vi "Get_Joystick.vi"(1 "Joystick_One":string="Pilot Controller", 2 "Joystick_Two":string="CoPilot Controller") -> (6 "Joystick_Out":T1)   [LabVIEW 2019]
uses:
  Joystick_Controls.ctl
  <vilib>/Rock Robotics/WPI/Utilities/WPI_GetSetVariantRefNum.vi
  <vilib>/Rock Robotics/WPI/Joystick/WPI_JoystickDeviceEnum.ctl
panel:
  in  "Joystick Controls":T1
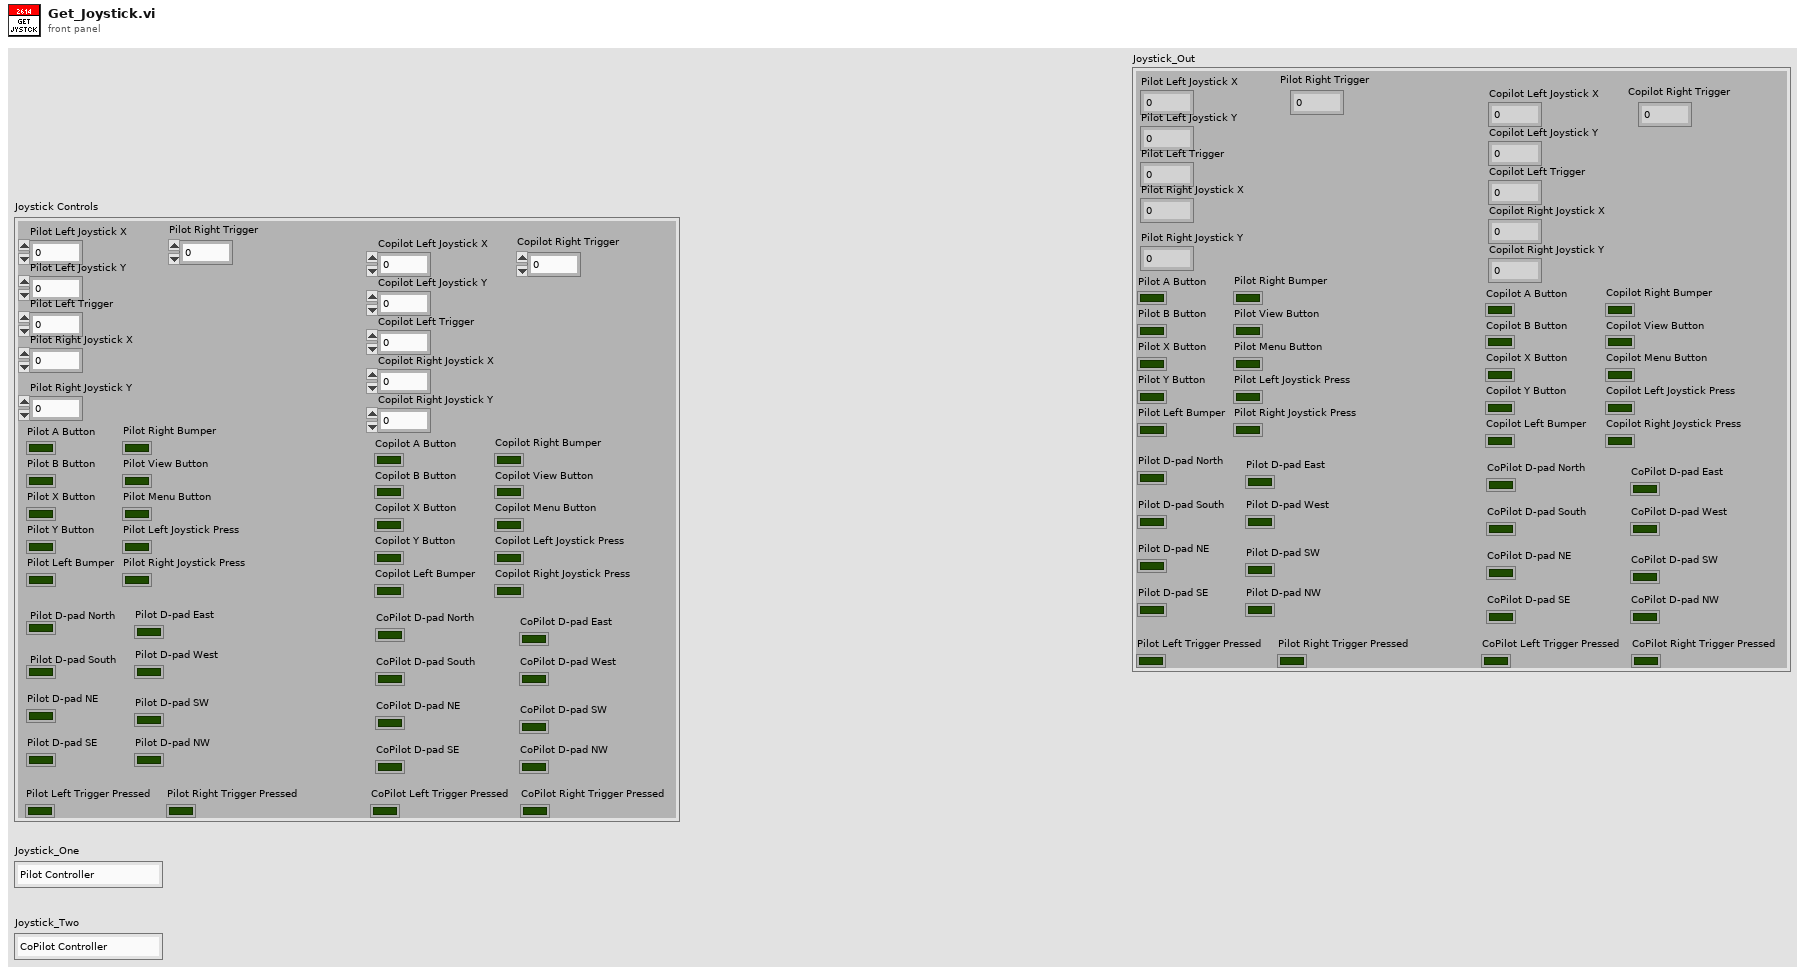
[diagram p1: front panel]
types:
  T1 = typedef "Joystick_Controls.ctl" = cluster{"Pilot Left Joystick X":dbl, "Pilot Left Joystick Y":dbl, "Pilot A Button":bool, "Pilot B Button":bool, "Pilot X Button":bool, "Pilot Y Button":bool, "Pilot Left Bumper":bool, "Pilot Right Bumper":bool, "Pilot View Button":bool, "Pilot Menu Button":bool, "Pilot Left Joystick Press":bool, "Pilot Right Joystick Press":bool, "Pilot Left Trigger":dbl, "Pilot Right Joystick X":dbl, "Pilot Right Joystick Y":dbl, "Pilot Right Trigger":dbl, "Copilot Left Joystick X":dbl, "Copilot Left Joystick Y":dbl, "Copilot A Button":bool, "Copilot B Button":bool, "Copilot X Button":bool, "Copilot Y Button":bool, "Copilot Left Bumper":bool, "Copilot Right Bumper":bool, "Copilot View Button":bool, "Copilot Menu Button":bool, "Copilot Left Joystick Press":bool, "Copilot Right Joystick Press":bool, "Copilot Left Trigger":dbl, "Copilot Right Joystick X":dbl, "Copilot Right Joystick Y":dbl, "Copilot Right Trigger":dbl, "Pilot D-pad North":bool, "Pilot D-pad South":bool, "Pilot D-pad East":bool, "Pilot D-pad West":bool, "Pilot D-pad NE ":bool, "Pilot D-pad SE":bool, "Pilot D-pad SW":bool, "Pilot D-pad NW":bool, "CoPilot D-pad North":bool, "CoPilot D-pad South":bool, "CoPilot D-pad East":bool, "CoPilot D-pad West":bool, "CoPilot D-pad NE":bool, "CoPilot D-pad SE":bool, "CoPilot D-pad SW":bool, "CoPilot D-pad NW":bool, "Pilot Left Trigger Pressed":bool, "Pilot Right Trigger Pressed":bool, "CoPilot Left Trigger Pressed":bool, "CoPilot Right Trigger Pressed":bool}
  T2 = typedef "WPI_JoystickDeviceEnum.ctl" = enum16{"USB 0", "USB 1", "USB 2", "USB 3", "USB 4", "USB 5"}
  T3 = typedef "WPI_Joystick Info.ctl" = cluster{"Device Name":string, "HID Type":T4, "XBox Type":T5, "Axes Count":i32, "Axes Types":T6[], "Button Count":i32, "POV Count":i32}
  T4 = typedef "WPI_JoystickHID Types.ctl" = enum16{"Not HID", "HID Joystick", "HID Gamepad", "HID Driving Wheel", "HID Flightstick", "HID First Person"}
  T5 = typedef "WPI_JoystickXBox Types.ctl" = enum16{"Not XBox", "XBox Unknown", "XBox Gamepad", "XBox Wheel", "XBox Arcade Stick", "XBox Flight Stick", "XBox Dance Pad", "XBox Guitar", "XBox Drum Kit", "XBox Arcade Pad"}
  T6 = typedef "WPI_JoystickAxis Types.ctl" = enum16{"X Axis", "Y Axis", "Z Axis", "RxAxis", "RyAxis", "RzAxis", "Slider", "POV", "None", "L X Axis", "L Y Axis", "L Trigger", "R Trigger", "R X Axis", "R Y Axis"}
  T7 = typedef "WPI_JoystickDevRef.ctl" = cluster{"Device":T2}
  T8 = cluster{"Axes[0]":dbl, "Axes[1]":dbl, "Axes[2]":dbl, "Axes[3]":dbl, "Axes[4]":dbl, "Axes[5]":dbl, "Axes[6]":dbl, "Axes[7]":dbl, "Axes[8]":dbl}
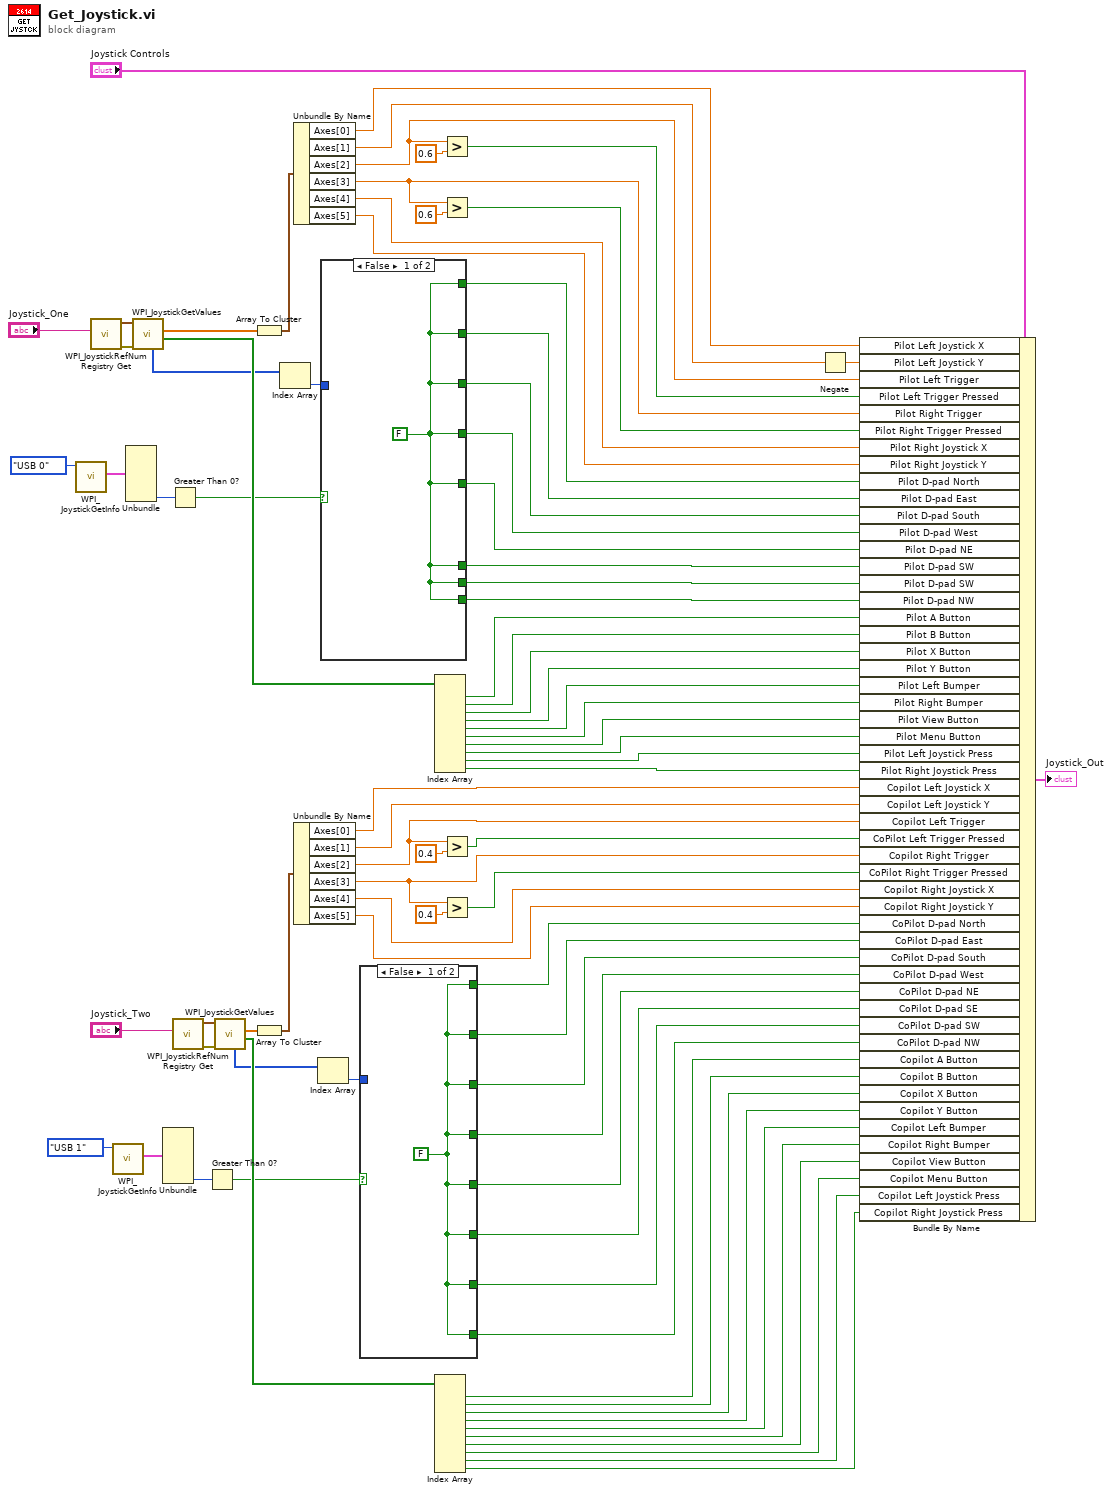
[diagram p0: block diagram]
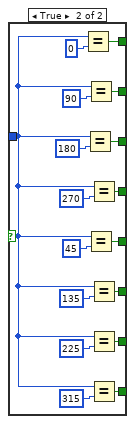
[diagram p2: hidden frame]
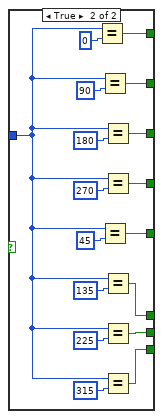
[diagram p3: hidden frame]
diagram:
  n1 = call <vilib>:"WPI_JoystickGetInfo.vi"("JoystickDevice"=WPI_JoystickDeviceEnum."USB 0") -> ("Joystick Info"=w7:T3)  [unwired: 9 in, 1 out]
  n2 = call <vilib>:"WPI_JoystickRefNum Registry Get.vi"("refnum name"="Joystick_One") -> ("error out"=w44:errorcluster, "JoystickDevRef"=w83:T7)  [unwired: 9 in]
  n3 = call <vilib>:"WPI_JoystickGetInfo.vi"("JoystickDevice"=WPI_JoystickDeviceEnum."USB 1") -> ("Joystick Info"=w3:T3)  [unwired: 9 in, 1 out]
  n4 = Unbundle(w7) -> ("POV Count"=w6:i32)  [unwired: 6 out]
  n5 = call <vilib>:"WPI_JoystickGetValues.vi"("error in (no error)"=w44, "JoystickDevRef"=w83) -> ("Buttons"=w76:bool[], "Axes"=w82:dbl[], "POVs"=w46:i16[])  [unwired: 5 in, 2 out]
  n6 = Unbundle(w3) -> ("POV Count"=w2:i32)  [unwired: 6 out]
  n7 = Greater Than 0?(x=w6) -> (x > 0?=w5:bool)
  n8 = call <vilib>:"WPI_JoystickRefNum Registry Get.vi"("refnum name"="Joystick_Two") -> ("error out"=w43:errorcluster, "JoystickDevRef"=w65:T7)  [unwired: 9 in]
  n9 = Greater Than 0?(x=w2) -> (x > 0?=w1:bool)
  n10 = call <vilib>:"WPI_JoystickGetValues.vi"("error in (no error)"=w43, "JoystickDevRef"=w65) -> ("Buttons"=w63:bool[], "Axes"=w64:dbl[], "POVs"=w45:i16[])  [unwired: 5 in, 2 out]
  n11 = Array To Cluster(array=w82) -> (cluster=w81:T8)
  n12 = Array To Cluster(array=w64) -> (cluster=w62:T8)
  n13 = Index Array(array=w46) -> (element=w33:i16)  [unwired: 1 in]
  n14 = Unbundle By Name(w81) -> ("Axes[0]"=w80:dbl, "Axes[1]"=w79:dbl, "Axes[2]"=w23:dbl, "Axes[3]"=w19:dbl, "Axes[4]"=w78:dbl, "Axes[5]"=w77:dbl)
  n15 = Unbundle By Name(w62) -> ("Axes[0]"=w61:dbl, "Axes[1]"=w60:dbl, "Axes[2]"=w16:dbl, "Axes[3]"=w13:dbl, "Axes[4]"=w59:dbl, "Axes[5]"=w58:dbl)
  n16 = Index Array(array=w45) -> (element=w24:i16)  [unwired: 1 in]
  n17 = case shown="False" w5 {
    tunnel: [w84 w101] -> w40
    tunnel: [w84 w100] -> w39
    tunnel: [w84 w99] -> w38
    tunnel: [w84 w98] -> w37
    tunnel: [w84 w97] -> w36
    tunnel: [w84 w96] -> w35
    tunnel: [w84 w95] -> w34
    tunnel: w33 -> [_ w85]
    tunnel: [w84 w86] -> w10
    frame False {
      w84 = FALSE
    }
    frame True {
      n18 = Equal?(x=w85, y=i16 0) -> (x = y?=w86:bool)
      n19 = Equal?(x=w85, y=i16 90) -> (x = y?=w101:bool)
      n20 = Equal?(x=w85, y=i16 45) -> (x = y?=w97:bool)
      n21 = Equal?(x=w85, y=i16 180) -> (x = y?=w100:bool)
      n22 = Equal?(x=w85, y=i16 270) -> (x = y?=w99:bool)
      n23 = Equal?(x=w85, y=i16 135) -> (x = y?=w96:bool)
      n24 = Equal?(x=w85, y=i16 225) -> (x = y?=w95:bool)
      n25 = Equal?(x=w85, y=i16 315) -> (x = y?=w98:bool)
    }
  }
  n26 = case shown="False" w1 {
    tunnel: [w102 w111] -> w32
    tunnel: [w102 w110] -> w31
    tunnel: [w102 w103] -> w30
    tunnel: [w102 w109] -> w29
    tunnel: [w102 w108] -> w28
    tunnel: [w102 w107] -> w27
    tunnel: [w102 w106] -> w26
    tunnel: [w102 w105] -> w25
    tunnel: w24 -> [_ w104]
    frame False {
      w102 = FALSE
    }
    frame True {
      n27 = Equal?(x=w104, y=i16 0) -> (x = y?=w111:bool)
      n28 = Equal?(x=w104, y=i16 180) -> (x = y?=w103:bool)
      n29 = Equal?(x=w104, y=i16 90) -> (x = y?=w110:bool)
      n30 = Equal?(x=w104, y=i16 45) -> (x = y?=w108:bool)
      n31 = Equal?(x=w104, y=i16 270) -> (x = y?=w109:bool)
      n32 = Equal?(x=w104, y=i16 135) -> (x = y?=w107:bool)
      n33 = Equal?(x=w104, y=i16 225) -> (x = y?=w106:bool)
      n34 = Equal?(x=w104, y=i16 315) -> (x = y?=w105:bool)
    }
  }
  n35 = Index Array(array=w76) -> (element #1=w75:bool, element #2=w74:bool, element #3=w73:bool, element #4=w72:bool, element #5=w71:bool, element #6=w70:bool, element #7=w69:bool, element #8=w68:bool, element #9=w67:bool, element #10=w66:bool)  [unwired: 10 in]
  n36 = Index Array(array=w63) -> (element #1=w57:bool, element #2=w56:bool, element #3=w55:bool, element #4=w54:bool, element #5=w52:bool, element #6=w53:bool, element #7=w51:bool, element #8=w50:bool, element #9=w49:bool, element #10=w48:bool)  [unwired: 10 in]
  n37 = Greater?(x=w23, y=0.6) -> (0:w21:bool)
  n38 = Greater?(x=w19, y=0.6) -> (0:w20:bool)
  n39 = Greater?(x=w16, y=0.4) -> (0:w17:bool)
  n40 = Greater?(x=w13, y=0.4) -> (0:w14:bool)
  n41 = Negate(x=w79) -> (-x=w9:dbl)
  n42 = Bundle By Name(cluster="Joystick Controls", "Pilot Left Joystick X"=w80, "Pilot Left Joystick Y"=w9, "Pilot Left Trigger"=w23, "Pilot Left Trigger Pressed"=w21, "Pilot Right Trigger"=w19, "Pilot Right Trigger Pressed"=w20, "Pilot Right Joystick X"=w78, "Pilot Right Joystick Y"=w77, "Pilot D-pad North"=w10, "Pilot D-pad East"=w40, "Pilot D-pad South"=w39, "Pilot D-pad West"=w38, "Pilot D-pad NE"=w36, "Pilot D-pad SW"=w35, "Pilot D-pad SW"=w34, "Pilot D-pad NW"=w37, "Pilot A Button"=w75, "Pilot B Button"=w74, "Pilot X Button"=w73, "Pilot Y Button"=w72, "Pilot Left Bumper"=w71, "Pilot Right Bumper"=w70, "Pilot View Button"=w69, "Pilot Menu Button"=w68, "Pilot Left Joystick Press"=w67, "Pilot Right Joystick Press"=w66, "Copilot Left Joystick X"=w61, "Copilot Left Joystick Y"=w60, "Copilot Left Trigger"=w16, "CoPilot Left Trigger Pressed"=w17, "Copilot Right Trigger"=w13, "CoPilot Right Trigger Pressed"=w14, "Copilot Right Joystick X"=w59, "Copilot Right Joystick Y"=w58, "CoPilot D-pad North"=w32, "CoPilot D-pad East"=w31, "CoPilot D-pad South"=w30, "CoPilot D-pad West"=w29, "CoPilot D-pad NE"=w28, "CoPilot D-pad SE"=w27, "CoPilot D-pad SW"=w26, "CoPilot D-pad NW"=w25, "Copilot A Button"=w57, "Copilot B Button"=w56, "Copilot X Button"=w55, "Copilot Y Button"=w54, "Copilot Left Bumper"=w52, "Copilot Right Bumper"=w53, "Copilot View Button"=w51, "Copilot Menu Button"=w50, "Copilot Left Joystick Press"=w49, "Copilot Right Joystick Press"=w48) -> (→"Joystick_Out":T1)
